vi "Fetch Multiple Record Multiple Channel.vi"   [LabVIEW 2012]
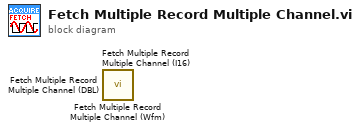
[diagram p0: block diagram]
diagram:
  n1 = call <userlib>:"Fetch Multiple Record Multiple Channel (Wfm).vi"() -> ()  [unwired: 8 in, 4 out]
  n2 = call <userlib>:"Fetch Multiple Record Multiple Channel (I16).vi"() -> ()  [unwired: 8 in, 4 out]
  n3 = call <userlib>:"Fetch Multiple Record Multiple Channel (DBL).vi"() -> ()  [unwired: 8 in, 4 out]
